vi "RPi WebDAV.vi"(8 "Error IN":errorcluster, 9 "RPi Sub-Dir":string="Sync", 10 "RPi IP":string="10.31.176.22", 11 "RIO Folder":path=path "c:/Closed_Data") -> (0 "Error OUT":errorcluster)   [LabVIEW 2013]
uses:
  <vilib>/WebDAVClient/Advanced/Put File.vi
  <vilib>/WebDAVClient/NI_WebDAV.lvlib
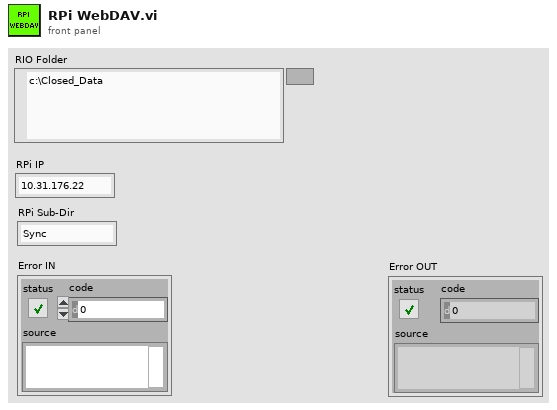
[diagram p1: front panel]
types:
  T1 = typedef "NI_WebDAV.lvlib/SessionHandle.ctl" = refnum<k1>
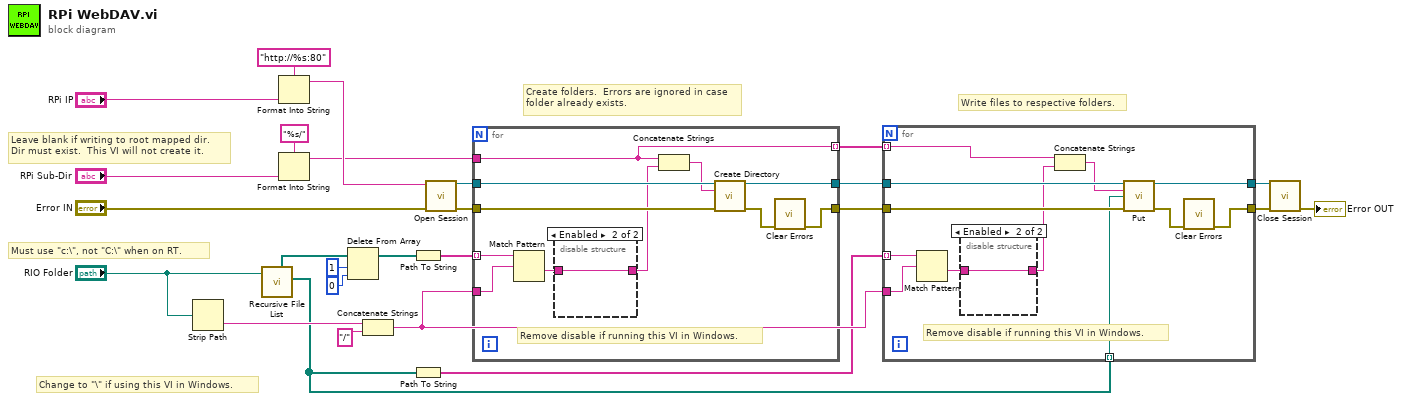
[diagram p0: block diagram]
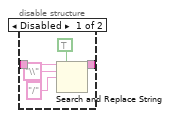
[diagram p2: hidden frame]
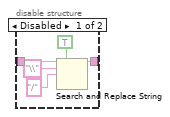
[diagram p3: hidden frame]
diagram:
  # "Leave blank if writing to root mapped dir.\nDir must exist.  This VI will not create it."
  # "Change to \"\\\" if using this VI in Windows."
  # "Must use \"c:\\\", not \"C:\\\" when on RT."
  # "Write files to respective folders."
  # "Create folders.  Errors are ignored in case\nfolder already exists."
  n1 = Strip Path(path="RIO Folder") -> (name=w21:string)  [unwired: 1 out]
  n2 = call <vilib>:"Recursive File List.vi"("Folder Path"="RIO Folder") -> ("All Files in Dir"=w19:path[], "All Folders"=w26:path[])  [unwired: 6 in, 3 out]
  n3 = Format Into String(format string="http://%s:80" ("file uri"), "RPi IP") -> (resulting string=w14:string)  [unwired: 2 in, 1 out]
  n4 = Format Into String(format string="%s/" ("file uri"), "RPi Sub-Dir") -> (resulting string=w2:string)  [unwired: 2 in, 1 out]
  n5 = Delete From Array(array=w26, length=1, index=0) -> (array with subset deleted=w23:path[])  [unwired: 1 out]
  n6 = Concatenate Strings(w21, "/" ("format string")) -> (w20:string)
  n7 = Path To String(path=w23) -> (string=w11:string[])
  n8 = Path To String(path=w19) -> (string=w8:string[])
  n9 = call <vilib>:"Open Session.vi"("host uri prefix"=w14, "error in (no error)"="Error IN") -> ("session handle out"=w12:T1, "error out"=w13:errorcluster)  [unwired: 12 in]
  n10 = for {
    tunnel: w13 -> [w36]
    tunnel: w12 -> [w35]
    tunnel: [w34] -> w10
    tunnel: [w33] -> w9
    tunnel: w11 -> [w32] mode=indexing
    tunnel: w20 -> [w31]
    tunnel: w2 -> [w27]
    tunnel: [w27] -> w1 mode=indexing
    # "Remove disable if running this VI in Windows."
    n11 = Match Pattern(string=w32, regular expression=w31) -> (after substring=w30:string)  [unwired: 1 in, 3 out]
    n12 = disable-structure shown="Enabled" {
      disable-tunnel: [w42 w43] -> w29
      disable-tunnel: w30 -> [w40 w43]
      frame Disabled {
        n13 = Search and Replace String(replace all?=TRUE ("replace all? (F)"), input string=w40, search string="\\", replace string="/" ("replace string (\"\")")) -> (result string=w42:string)  [unwired: 4 in, 3 out]
      }
      frame Enabled {
      }
    }
    n14 = Concatenate Strings(w27, w29) -> (w28:string)
    n15 = call <vilib>:"Create Directory.vi"("session handle"=w35, "relative uri"=w28, "error in (no error)"=w36) -> ("session handle out"=w34:T1, "error out"=w37:errorcluster)  [unwired: 11 in]
    n16 = call <vilib>:"Clear Errors.vi"("error in (no error)"=w37) -> ("error out"=w33:errorcluster)  [unwired: 6 in]
  }
  n17 = for {
    tunnel: w9 -> [w54]
    tunnel: w10 -> [w53]
    tunnel: [w52] -> w7
    tunnel: [w51] -> w6
    tunnel: w8 -> [w50] mode=indexing
    tunnel: w20 -> [w49]
    tunnel: w19 -> [w48] mode=indexing
    tunnel: w1 -> [w46] mode=indexing
    # "Remove disable if running this VI in Windows."
    n18 = Match Pattern(string=w50, regular expression=w49) -> (after substring=w47:string)  [unwired: 1 in, 3 out]
    n19 = disable-structure shown="Enabled" {
      disable-tunnel: [w60 w61] -> w45
      disable-tunnel: w47 -> [w58 w61]
      frame Disabled {
        n20 = Search and Replace String(replace all?=TRUE ("replace all? (F)"), input string=w58, search string="\\", replace string="/" ("replace string (\"\")")) -> (result string=w60:string)  [unwired: 4 in, 3 out]
      }
      frame Enabled {
      }
    }
    n21 = Concatenate Strings(w46, w45) -> (w44:string)
    n22 = call-poly <vilib>:"Put.vi"("session handle"=w53, "relative uri"=w44, "local file path"=w48, "error in (no error)"=w54) -> ("session handle out"=w52:T1, "error out"=w55:errorcluster)  [unwired: 9 in, 1 out]
    n23 = call <vilib>:"Clear Errors.vi"("error in (no error)"=w55) -> ("error out"=w51:errorcluster)  [unwired: 6 in]
  }
  n24 = call <vilib>:"Close Session.vi"("session handle"=w7, "error in (no error)"=w6) -> ("error out"=→"Error OUT":errorcluster)  [unwired: 13 in]
